vi "Create new and initialise.vi"(8 "error in (no error)":errorcluster, 11 "Serialisation Type":T1) -> (0 "error out":errorcluster, 3 "EventsParent out":refnum<class "Events.lvclass">)   [LabVIEW 2020, in "wamplv.lvlib" / "Events.lvclass"]
uses:
  Events.lvclass
  Events.lvclass/Events.ctl
  JsonEvents/JsonEvents.lvclass
  MsgPackEvents/MsgPackEvents.lvclass
  C:/local/wamplv/Private/Events/EventsParent/Events.lvclass
  C:/local/wamplv/Private/Events/JsonEvents/JsonEvents.lvclass
  C:/local/wamplv/Private/Events/MsgPackEvents/MsgPackEvents.lvclass
  WAMP Client/API/TypeDefs/Serialisation.ctl
  WAMP Client/WAMP Client.lvclass
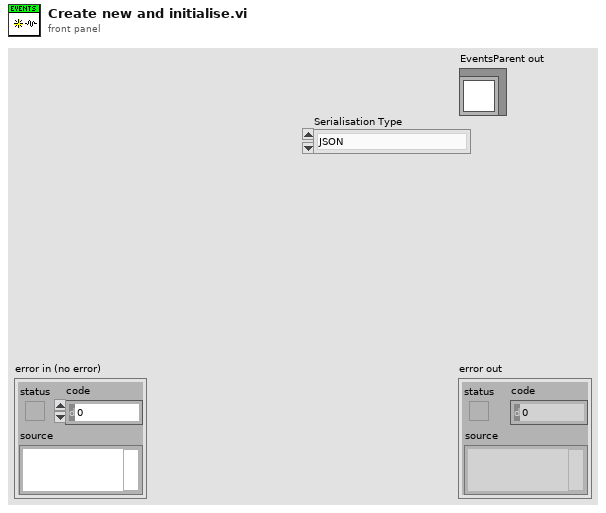
[diagram p1: front panel]
types:
  T1 = typedef "wamplv.lvlib/WAMP Client.lvclass/Serialisation.ctl" = enum16{"JSON", "MessagePack"}
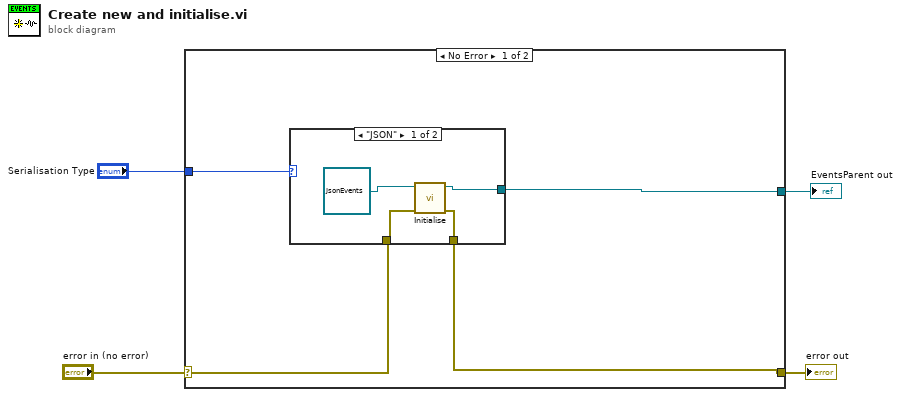
[diagram p0: block diagram]
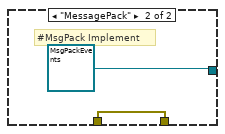
[diagram p2: hidden frame]
diagram:
  n1 = case shown="No Error" "error in (no error)" {
    selector: "error in (no error)" -> [w6 w15]
    tunnel: [w5 w15] -> w3
    tunnel: [w7 _] -> w2
    tunnel: "Serialisation Type" -> [w8 _]
    frame No Error {
      n2 = case shown="\"JSON\"" w8 {
        tunnel: [w11 refnum<class "MsgPackEvents.lvclass"> refnum ("wamplv.lvlib:MsgPackEvents.lvclass")] -> w7
        tunnel: w6 -> [w10 w14]
        tunnel: [w9 w14] -> w5
        frame "JSON" {
          n3 = call-dynamic "Initialise.vi"("error in (no error)"=w10, "JsonEvents in"=refnum<class "JsonEvents.lvclass"> refnum ("wamplv.lvlib:JsonEvents.lvclass")) -> ("error out"=w9:errorcluster, "JsonEvents out"=w11:refnum<class "JsonEvents.lvclass">)  [unwired: 8 in]
        }
        frame "MessagePack" {
          # "#MsgPack Implement"
        }
      }
    }
    frame Error {
    }
  }
  "error out" <- w3
  "EventsParent out" <- w2
